vi "CRYDB Insert Into ItemTable.vi"(0 "connection reference":T1, 3 "error in":errorcluster) -> (7 "connection reference out":T1, 8 "Item_ID":i32, 10 "error out":errorcluster)   [LabVIEW 2013]
uses:
  <vilib>/addons/database/Connection.llb/Conn ObjectReference.ctl
  <vilib>/addons/database/Auxilliary.llb/DB Tools Column Info.ctl
  <vilib>/addons/database/Auxilliary.llb/DB Tools DataTypes.ctl
  Data/CRYData & result stacks global.vi
  <vilib>/addons/database/Connection.llb/Conn Execute.vi
  <vilib>/addons/database/Recordset.llb/Rec Fetch Recordset Data (R).vi
  <vilib>/addons/database/Recordset.llb/Rec Destroy - Connection.vi
  <vilib>/addons/database/_DB Variant To Data/Database Variant To Data.xnode
  <vilib>/addons/database/NI_Database_API.lvlib
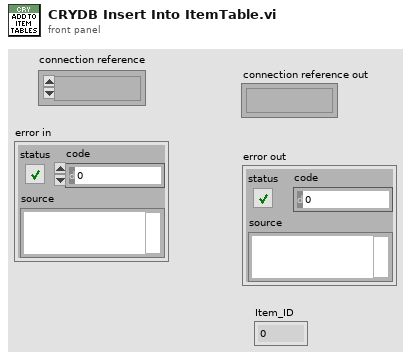
[diagram p1: front panel]
types:
  T1 = typedef "NI_Database_API.lvlib/Conn ObjectReference.ctl" = refnum<k1>
  T2 = typedef "NI_Database_API.lvlib/DB Tools Column Info.ctl" = cluster{"column name":string, "data type":T3, "size":i32, "allow null?":bool}
  T3 = typedef "NI_Database_API.lvlib/DB Tools DataTypes.ctl" = enum16{"String", "Long (I32)", "Single (SGL)", "Double (DBL)", "Date/Time", "Binary"}
  T4 = cluster{"Item_ID":u32, "Serial_No":string, "Lot_No":string, "Item_Des":string}
  T5 = typedef "NI_Database_API.lvlib/Rec ObjectReference.ctl" = refnum<k1>
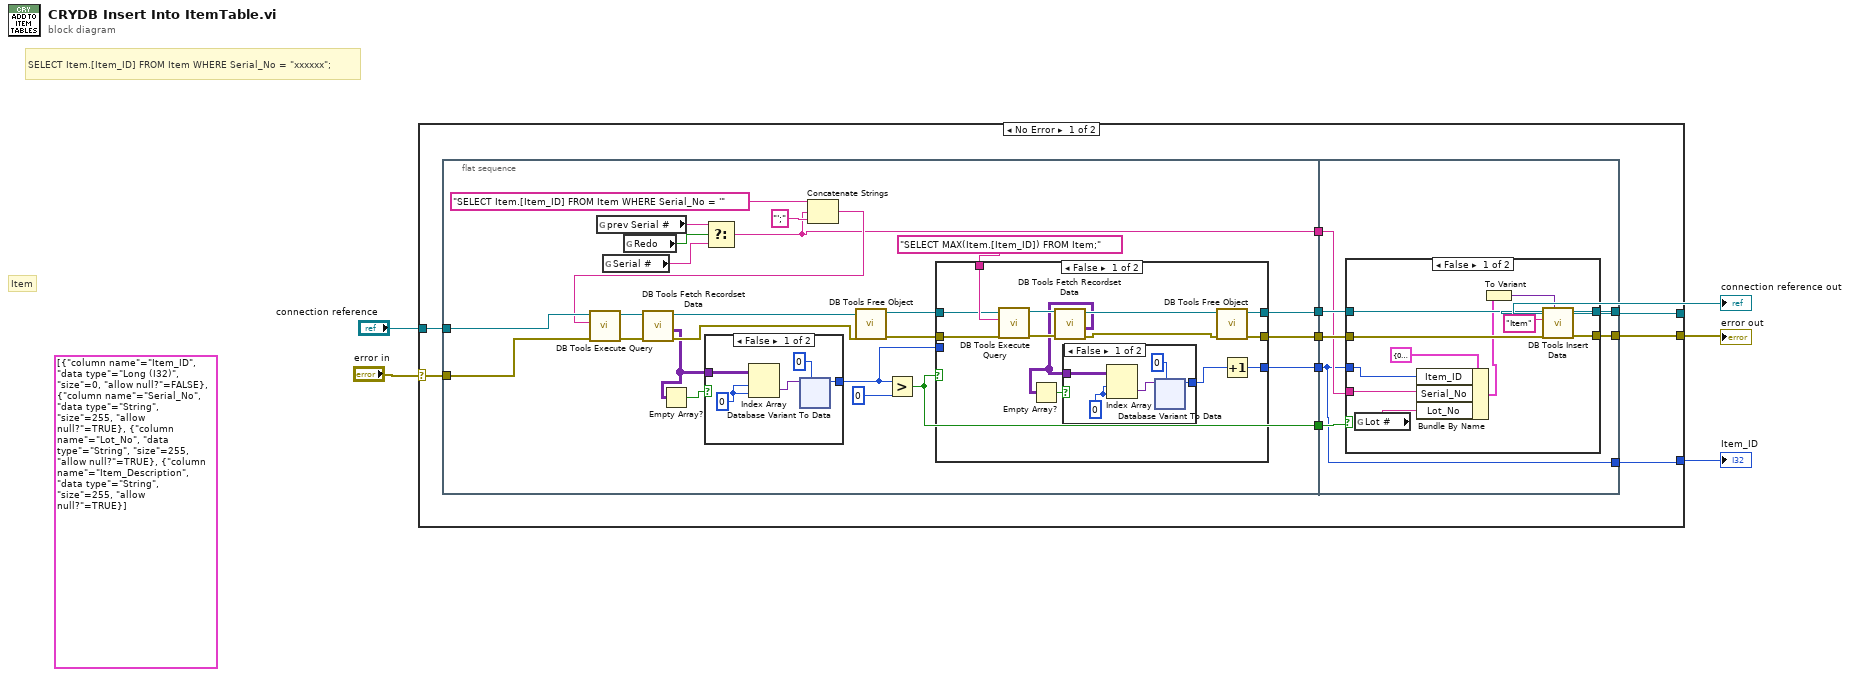
[diagram p0: block diagram]
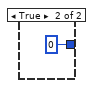
[diagram p2: hidden frame]
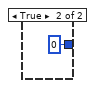
[diagram p3: hidden frame]
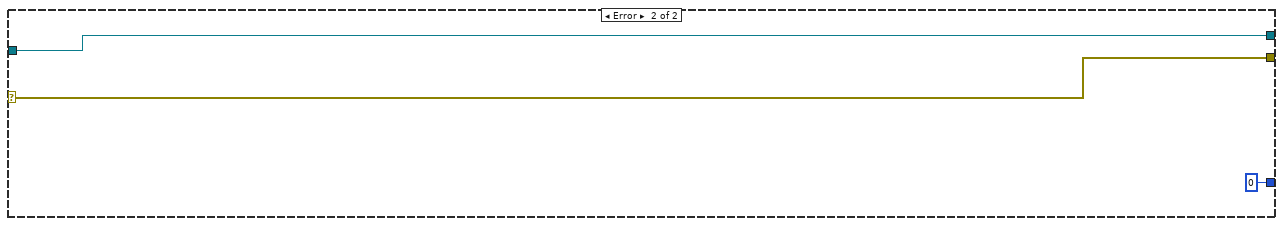
[diagram p6: hidden frame]
diagram:
  (unwired) T2[] [{"column name"="Item_ID", "data type"=enum."Long (I32)", "size"=0, "allow null?"=FALSE}, {"column name"="Serial_No", "data type"=enum."String", "size"=255, "allow null?"=TRUE}, {"column name"="Lot_No", "data type"=enum."String", "size"=255, "allow null?"=TRUE}, {"column name"="Item_Description", "data type"=enum."String", "size"=255, "allow null?"=TRUE}] ("column information")
  # "SELECT Item.[Item_ID] FROM Item WHERE Serial_No = \"xxxxxx\";"
  # "Item"
  n1 = case shown="No Error" "error in" {
    selector: "error in" -> [w13 w153]
    tunnel: "connection reference" -> [w15 w154]
    tunnel: [w11 w154] -> w2
    tunnel: [w10 w153] -> w3
    tunnel: [w6 0 ("data")] -> w1
    frame No Error {
      n2 = flat-sequence {
        tunnel: w15 -> [w39]
        tunnel: [w22] -> w14
        tunnel: w13 -> [w35]
        tunnel: [w21] -> w12
        tunnel: [w20] -> w9
        tunnel: [w19] -> w8
        tunnel: [w18] -> w7
        tunnel: w14 -> [w138]
        tunnel: w12 -> [w137]
        tunnel: [w136] -> w11
        tunnel: [w135] -> w10
        tunnel: w9 -> [w134]
        tunnel: w8 -> [w132]
        tunnel: w7 -> [w133]
        tunnel: [w132] -> w6
        frame #0 {
          n3 = global read "CRYData & result stacks global.vi" "prev Serial #"() -> (w32:string)
          n4 = global read "CRYData & result stacks global.vi" "Serial #"() -> (w31:string)
          n5 = global read "CRYData & result stacks global.vi" "Redo"() -> (w30:bool)
          n6 = Select(t=w32, s=w30, f=w31) -> (s? t:f=w18:string)
          n7 = Concatenate Strings("SELECT Item.[Item_ID] FROM Item WHERE Serial_No = '" ("SQL query"), w18, "';" ("string")) -> (w27:string)
          n8 = call-poly <vilib>:"DB Tools Execute Query.vi"("error in (no error)"=w35, "SQL query"=w27, "connection reference"=w39) -> ("error out"=w34:errorcluster, "recordset reference"=w38:T5)  [unwired: 5 in]
          n9 = call-poly <vilib>:"DB Tools Fetch Recordset Data.vi"("error in (no error)"=w34, "recordset reference"=w38) -> ("error out"=w33:errorcluster, "recordset data"=w17:variant[][], "recordset reference out"=w37:T5)  [unwired: 3 in]
          n10 = Empty Array?(array=w17) -> (empty?=w16:bool)
          n11 = case shown="False" w16 {
            tunnel: w17 -> [w44 _]
            tunnel: [w41 0 ("data")] -> w26
            frame False {
              w43 = 0 ("disabled index (col)")
              n12 = Index Array(array=w44, index (row)=w43, index (col)=w43) -> (element=w40:variant)
              n13 = xnode "Database Variant To Data"("database variant"=w40, "type"=0) -> ("data"=w41:i32)  [unwired: 1 in, 1 out]
            }
            frame True {
            }
          }
          n14 = call-poly <vilib>:"DB Tools Free Object.vi"("error in (no error)"=w33, "recordset reference"=w37) -> ("error out"=w24:errorcluster, "connection reference"=w25:T1)  [unwired: 8 in]
          n15 = Greater?(x=w26, y=0) -> (0:w20:bool)
          n16 = case shown="False" w20 {
            tunnel: w26 -> [_ w131]
            tunnel: w25 -> [w89 w130]
            tunnel: w24 -> [w88 w129]
            tunnel: "SELECT MAX(Item.[Item_ID]) FROM Item;" ("SQL query") -> [w90 _]
            tunnel: [w85 w131] -> w19
            tunnel: [w82 w130] -> w22
            tunnel: [w81 w129] -> w21
            frame False {
              n17 = call-poly <vilib>:"DB Tools Execute Query.vi"("error in (no error)"=w88, "SQL query"=w90, "connection reference"=w89) -> ("error out"=w86:errorcluster, "recordset reference"=w87:T5)  [unwired: 5 in]
              n18 = call-poly <vilib>:"DB Tools Fetch Recordset Data.vi"("error in (no error)"=w86, "recordset reference"=w87) -> ("error out"=w83:errorcluster, "recordset data"=w78:variant[][], "recordset reference out"=w84:T5)  [unwired: 3 in]
              n19 = Empty Array?(array=w78) -> (empty?=w80:bool)
              n20 = case shown="False" w80 {
                tunnel: w78 -> [w95 _]
                tunnel: [w92 0 ("data")] -> w79
                frame False {
                  w94 = 0 ("disabled index (col)")
                  n21 = Index Array(array=w95, index (row)=w94, index (col)=w94) -> (element=w91:variant)
                  n22 = xnode "Database Variant To Data"("database variant"=w91, "type"=0) -> ("data"=w92:i32)  [unwired: 1 in, 1 out]
                }
                frame True {
                }
              }
              n23 = call-poly <vilib>:"DB Tools Free Object.vi"("error in (no error)"=w83, "recordset reference"=w84) -> ("error out"=w81:errorcluster, "connection reference"=w82:T1)  [unwired: 8 in]
              n24 = Increment(x=w79) -> (x+1=w85:i32)
            }
            frame True {
            }
          }
        }
        frame #1 {
          n25 = case shown="False" w134 {
            tunnel: w138 -> [w149 w151]
            tunnel: w137 -> [w147 w150]
            tunnel: [w145 w151] -> w136
            tunnel: [w144 w150] -> w135
            tunnel: w132 -> [w142 _]
            tunnel: w133 -> [w141 _]
            frame False {
              n26 = global read "CRYData & result stacks global.vi" "Lot #"() -> (w140:string)
              n27 = Bundle By Name(cluster=T4 {"Item_ID"=0, "Serial_No"="", "Lot_No"="", "Item_Des"=""} ("Item Table Out"), "Item_ID"=w142, "Serial_No"=w141, "Lot_No"=w140) -> (w139:T4)
              n28 = To Variant(anything=w139) -> (Variant=w146:variant)
              n29 = call <vilib>:"DB Tools Insert Data.vi"("data"=w146, "error in (no error)"=w147, "table"="Item", "connection reference"=w149) -> ("error out"=w144:errorcluster, "connection reference out"=w145:T1)  [unwired: 6 in]
            }
            frame True {
            }
          }
        }
      }
    }
    frame Error {
    }
  }
  "connection reference out" <- w2
  "error out" <- w3
  "Item_ID" <- w1
